vi "draw a line -- array -- complex.vi"(10 "Array":cdb[](array[numeric])) -> (3 "output cluster":cluster{dbl[], dbl[]})   [LabVIEW 2018]
uses:
  generate linear region --complex -- win cen.vi
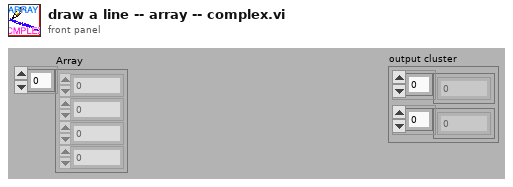
[diagram p1: front panel]
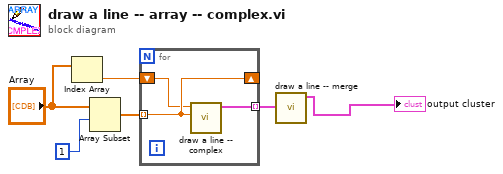
[diagram p0: block diagram]
diagram:
  n1 = Index Array(array="Array") -> (element=w5:cdb)  [unwired: 1 in]
  n2 = Array Subset(array="Array", index=1) -> (w1:cdb[])  [unwired: 1 in]
  n3 = for {
    tunnel: w1 -> [w9] mode=indexing
    shift-right: [w9] -> _
    shift-left: w5 -> [w7]
    tunnel: [w8] -> w6 mode=indexing
    n4 = call "draw a line -- complex.vi"("x1"=w9, "x0"=w7) -> ("output cluster"=w8:cluster{dbl[], dbl[]})  [unwired: 9 in]
  }
  n5 = call "draw a line -- merge.vi"("Array"=w6) -> ("output cluster"=→"output cluster":cluster{dbl[], dbl[]})  [unwired: 10 in]
